vi "WriteFileType.vi"(8 "error in (no error)":errorcluster, 10 "File Type":T1, 11 "object in":refnum<class "DataType.lvclass">) -> (0 "error out":errorcluster, 3 "object out":refnum<class "DataType.lvclass">)   [LabVIEW 2024, in "DataType.lvclass"]
uses:
  <resource>/Framework/Providers/Open_GDS/ClassProviders/Provider_LvNativeClass/Templates/NativeBaseTemplate/NativeBaseTemplate.lvclass/NativeBaseTemplate.ctl
  DataType.lvclass
  DataType.lvclass/DataType.ctl
  Support/Type Def/File Type.ctl
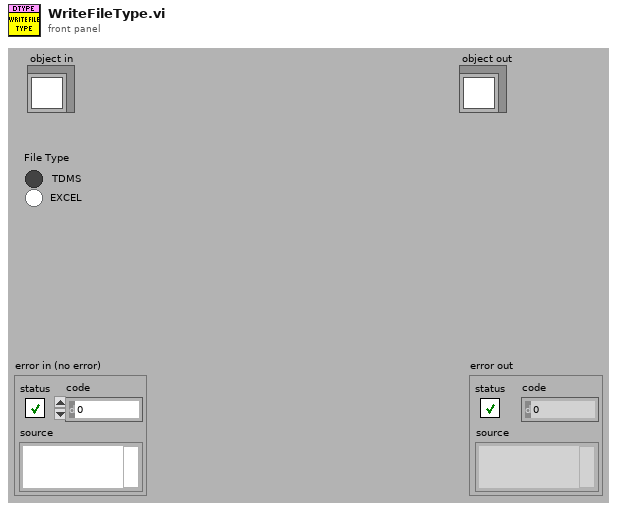
[diagram p1: front panel]
types:
  T1 = typedef "File Type.ctl" = enum32{"TDMS", "EXCEL"}
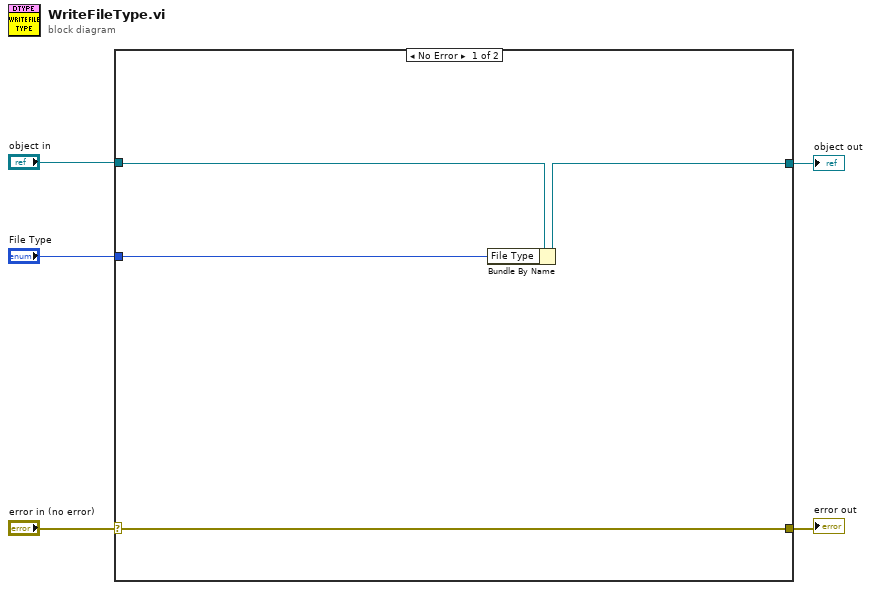
[diagram p0: block diagram]
diagram:
  n1 = case shown="No Error" "error in (no error)" {
    selector: "error in (no error)" -> [w8 w11]
    tunnel: [w8 w11] -> w4
    tunnel: [w6 w10] -> w2
    tunnel: "object in" -> [w7 w10]
    tunnel: "File Type" -> [w9 _]
    frame No Error {
      n2 = Bundle By Name(cluster=w7, "File Type"=w9) -> (w6:refnum<class "DataType.lvclass">)
    }
    frame Error {
    }
  }
  "error out" <- w4
  "object out" <- w2
